vi "Find Graves.vi"(8 "Error In":errorcluster, 11 "VI In":refnum<vi>) -> (0 "Error Out":errorcluster, 2 "Graves":refnum<vi>[](array[refnum]), 3 "VI Out":refnum<vi>)   [LabVIEW 2017, in "Toolkit.lvlib"]
doc: "Finds all graves in the block diagram of a VI."
uses:
  Toolkit.lvlib
  <vilib>/Utility/traverseref.llb/TRef TravTarget.ctl
  <vilib>/Utility/traverseref.llb/VI Scripting - Traverse.lvlib
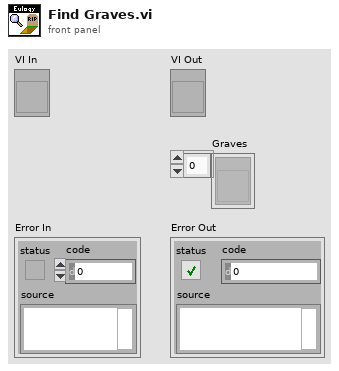
[diagram p1: front panel]
types:
  T1 = typedef "TRef TravTarget.ctl" = enum16{"FP", "BD", "Other"}
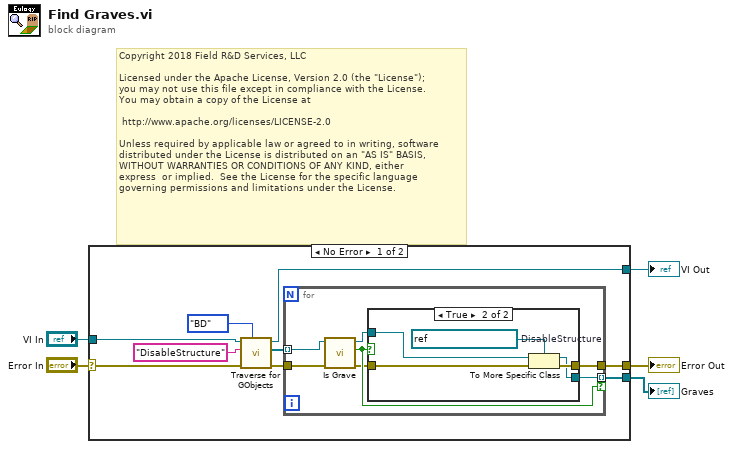
[diagram p0: block diagram]
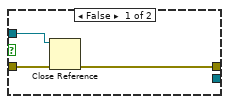
[diagram p2: hidden frame]
diagram:
  # "Copyright 2018 Field R&D Services, LLC\n\nLicensed under the Apache License, Version 2.0 (the \"License\");\nyou may not use this file except in compliance with the License.\nYou may obtain a copy of the License at\n\n\thttp://www.apache.org/licenses/LICENSE-2.0\n\nUnless required by applicable law or agreed to in writing, software\ndistributed under the License is distributed on an \"AS IS\" BASIS,\nWITHOUT WARRANTIES OR CONDITIONS OF ANY KIND, either \nexpress  or implied.  See the License for the specific language \ngoverning permissions and limitations under the License."
  n1 = case shown="No Error" "Error In" {
    selector: "Error In" -> [w6 w30]
    tunnel: "VI In" -> [w12 w31]
    tunnel: [w9 w30] -> w4
    tunnel: [w8 w31] -> w3
    tunnel: [w7 _] -> w2
    frame No Error {
      n2 = call <vilib>:"Traverse for GObjects.vi"("Traverse Target"=TRef_TravTarget."BD", "error in (no error)"=w6, "Class Name"="DisableStructure", "VI Refnum"=w12) -> ("error out"=w11:errorcluster, "References"=w10:refnum<vi>[], "dup VI Refnum"=w8:refnum<vi>)  [unwired: 4 in, 1 out]
      n3 = for {
        tunnel: w11 -> [w21]
        tunnel: w10 -> [w20] mode=indexing
        tunnel: [w18] -> w7 mode=indexing if=w17
        tunnel: [w15] -> w9
        n4 = call "Is Grave.vi"("Error In"=w21, "GObject In"=w20) -> ("Error Out"=w16:errorcluster, "Grave?"=w17:bool, "GObject Out"=w19:refnum<vi>)  [unwired: 7 in]
        n5 = case shown="True" w17 {
          tunnel: w19 -> [w24 w27]
          tunnel: [_ w26] -> w18
          tunnel: w16 -> [w23 w29]
          tunnel: [w22 w28] -> w15
          frame False {
            n6 = Close Reference(reference=w24, error in (no error)=w23) -> (error out=w22:errorcluster)
          }
          frame True {
            w25 = refnum<vi> refnum  # DisableStructure
            n7 = To More Specific Class(target class=w25, reference=w27, error in=w29) -> (specific class reference=w26:refnum<vi>, error out=w28:errorcluster)
          }
        }
      }
    }
    frame Error {
    }
  }
  "Error Out" <- w4
  "VI Out" <- w3
  "Graves" <- w2
